vi "Test Refresh Existing Rectangle Settings.vi"(8 "error in (no error)":errorcluster) -> (0 "error out":errorcluster)   [LabVIEW 2019]
uses:
  Setting Database/Setting Database.lvclass
  C:/Program Files (x86)/National Instruments/LabVIEW 2019/vi.lib/JKI/JKI SMO/SMO/SMO.lvclass
  ObjectSettings/ObjectSettings.lvclass/ObjectSettings.ctl
  ObjectSettings/Accessors/Read Enabled.vi
  ObjectSettings/Accessors/Write Enabled.vi
  Rectangle Settings/Rectangle Settings.lvclass
  C:/Users/Albro/Documents/GitHub/AFM-Lithography/lvsrc/Classes/Settings/ObjectSettings/ObjectSettings.lvclass
  <vilib>/addons/_JKI Toolkits/Caraya/classes/Assert/Assert Equal Value_Variant.vi
  <vilib>/addons/_JKI Toolkits/Caraya/classes/Test/Test.lvclass
  <vilib>/addons/_JKI Toolkits/Caraya/classes/Assert/Assert.lvclass
  <vilib>/JKI/JKI SMO/SMO/SMO.lvclass
  <vilib>/LabVIEW Open Source Project/Unicity/RandomStringGenerator/RandomStringGenerator.lvclass
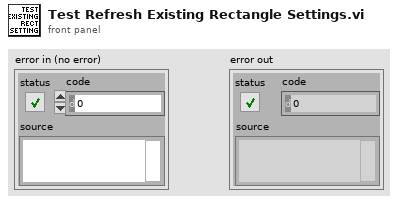
[diagram p1: front panel]
types:
  T1 = typedef "Setting Database.lvclass/PublicEvents--Cluster.ctl" = cluster{"NewActivePath":refnum<user-event>, "PathsUpdated":refnum<user-event>, "RectanglesUpdated":refnum<user-event>, "NewActiveRectangle":refnum<user-event>, "NewActiveFunnel":refnum<user-event>, "FunnelsUpdated":refnum<user-event>, "NewActiveDot":refnum<user-event>, "DotsUpdated":refnum<user-event>}
  T2 = typedef "Setting Database.lvclass/PrivateEvents--Setting Database.Refresh.ctl" = cluster{"Paths":string[], "Rectangles":string[], "Funnels":string[], "Dots":string[]}
  T3 = typedef "Setting Database.lvclass/PublicEvents--Setting Database.NewActiveRectangle.ctl" = refnum<class "Rectangle Settings.lvclass">
  T4 = typedef "Setting Database.lvclass/PublicEvents--Setting Database.RectanglesUpdated.ctl" = refnum<class "Rectangle Settings.lvclass">[]
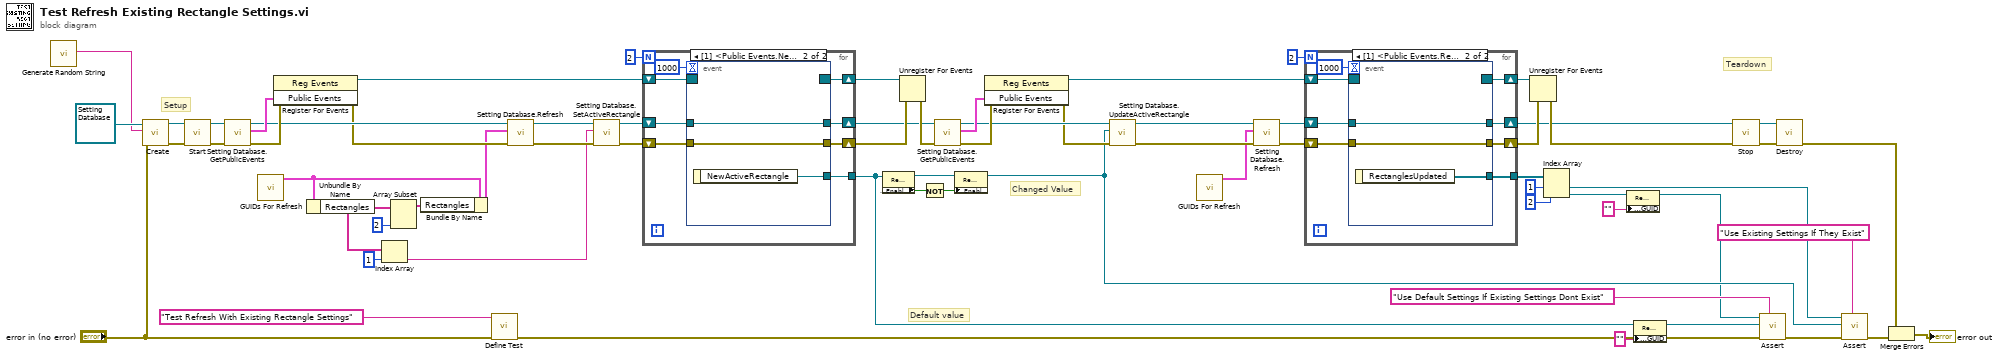
[diagram p0: block diagram]
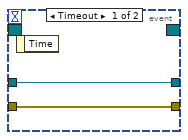
[diagram p2: hidden frame]
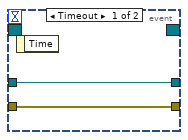
[diagram p3: hidden frame]
diagram:
  # "Changed Value"
  # "Default value"
  # "Teardown"
  # "Setup"
  n1 = call <vilib>:"Generate Random String.vi"() -> ("Random String"=w1:string)  [unwired: 11 in]
  n2 = call <vilib>:"Create.vi"("error in (no error)"="error in (no error)", "Subsystem Name (optional)"=w1, "SMO"=refnum<class "Setting Database.lvclass"> refnum ("Setting Database.lvclass")) -> ("error out"=w66:errorcluster, "SMO out"=w58:refnum<class "Setting Database.lvclass">)  [unwired: 6 in, 1 out]
  n3 = call <vilib>:"Start.vi"("error in (no error)"=w66, "SMO"=w58) -> ("error out"=w65:errorcluster, "SMO out"=w57:refnum<class "Setting Database.lvclass">)  [unwired: 8 in]
  n4 = call "Setting Database.GetPublicEvents.vi"("error in (no error)"=w65, "Setting Database"=w57) -> ("error out"=w63:errorcluster, "Public Events"=w53:T1, "Setting Database out"=w51:refnum<class "Setting Database.lvclass">)  [unwired: 7 in]
  n5 = call "GUIDs For Refresh.vi"() -> ("Initialize"=w13:T2)  [unwired: 11 in]
  n6 = register-events(error in=w63, w53) -> (reference out=w54:refnum<event-registration>, error out=w50:errorcluster)  [unwired: 1 in]
  n7 = Unbundle By Name(w13) -> ("Rectangles"=w11:string[])
  n8 = Index Array(array=w11, index=1) -> (element=w9:string)
  n9 = Array Subset(array=w11, length=2) -> (w14:string[])  [unwired: 1 in]
  n10 = Bundle By Name(cluster=w13, "Rectangles"=w14) -> (w12:T2)
  n11 = call <vilib>:"Define Test.vi"("error in (no error)"="error in (no error)", "Label (VI Title)"="Test Refresh With Existing Rectangle Settings") -> ("error out"=w25:errorcluster)  [unwired: 8 in, 1 out]
  n12 = call "Setting Database.Refresh.vi"("error in (no error)"=w50, "Initialize"=w12, "Setting Database"=w51) -> ("error out"=w21:errorcluster, "Setting Database out"=w24:refnum<class "Setting Database.lvclass">)  [unwired: 7 in]
  n13 = call "Setting Database.SetActiveRectangle.vi"("error in (no error)"=w21, "SetActiveRectangle"=w9, "Setting Database"=w24) -> ("error out"=w22:errorcluster, "Setting Database out"=w23:refnum<class "Setting Database.lvclass">)  [unwired: 7 in]
  n14 = for {
    N: 2 -> [_]
    tunnel: [w68] -> w6
    shift-right: [w74] -> w55
    shift-left: w54 -> [w72]
    shift-right: [w75] -> w45
    shift-left: w22 -> [w70]
    shift-right: [w71] -> w41
    shift-left: w23 -> [w69]
    n15 = event shown="[1] <Public Events.NewActiveRectangle>: User Event" {
      selector: w72 -> [_ _]
      dyn-events: [_ _] -> w74
      timeout: 1000 -> [_ _]
      tunnel: [w77 w80] -> w75
      tunnel: w70 -> [w77 w80]
      tunnel: w69 -> [w76 w79]
      tunnel: [w76 w79] -> w71
      tunnel: [_ w78] -> w68
      event Timeout {
        n16 = event-data() -> ()  [unwired: 1 in, 1 out]
      }
      event User Event {
        n17 = event-data() -> ("NewActiveRectangle"=w78:T3)  [unwired: 1 in]
      }
    }
  }
  n18 = property on="Property Node" class="Rectangle Settings.lvclass"(reference=w6) -> (reference out=w47:T3, "Accessors:Enabled"=w49:bool)  [unwired: 1 in, 1 out]
  n19 = Unregister For Events(event registration refnum=w55, error in=w45) -> (error out=w42:errorcluster)
  n20 = Not(x=w49) -> (.not. x?=w48:bool)
  n21 = call "Setting Database.GetPublicEvents.vi"("error in (no error)"=w42, "Setting Database"=w41) -> ("error out"=w43:errorcluster, "Public Events"=w44:T1, "Setting Database out"=w20:refnum<class "Setting Database.lvclass">)  [unwired: 7 in]
  n22 = property on="Property Node" class="Rectangle Settings.lvclass"(reference=w47, "Accessors:Enabled"=w48) -> (reference out=w16:T3)  [unwired: 1 in, 1 out]
  n23 = register-events(error in=w43, w44) -> (reference out=w38:refnum<event-registration>, error out=w17:errorcluster)  [unwired: 1 in]
  n24 = call "Setting Database.UpdateActiveRectangle.vi"("error in (no error)"=w17, "UpdateActiveRectangle"=w16, "Setting Database"=w20) -> ("error out"=w18:errorcluster, "Setting Database"=w19:refnum<class "Setting Database.lvclass">)  [unwired: 7 in]
  n25 = call "GUIDs For Refresh.vi"() -> ("Initialize"=w8:T2)  [unwired: 11 in]
  n26 = call "Setting Database.Refresh.vi"("error in (no error)"=w18, "Initialize"=w8, "Setting Database"=w19) -> ("error out"=w40:errorcluster, "Setting Database out"=w39:refnum<class "Setting Database.lvclass">)  [unwired: 7 in]
  n27 = for {
    N: 2 -> [_]
    tunnel: [w81] -> w33
    shift-right: [w87] -> w37
    shift-left: w38 -> [w85]
    shift-right: [w88] -> w36
    shift-left: w40 -> [w83]
    shift-right: [w84] -> w34
    shift-left: w39 -> [w82]
    n28 = event shown="[1] <Public Events.RectanglesUpdated>: User Event" {
      selector: w85 -> [_ _]
      dyn-events: [_ _] -> w87
      timeout: 1000 -> [_ _]
      tunnel: [w90 w93] -> w88
      tunnel: w83 -> [w90 w93]
      tunnel: w82 -> [w89 w92]
      tunnel: [w89 w92] -> w84
      tunnel: [_ w91] -> w81
      event Timeout {
        n29 = event-data() -> ()  [unwired: 1 in, 1 out]
      }
      event User Event {
        n30 = event-data() -> ("RectanglesUpdated"=w91:T4)  [unwired: 1 in]
      }
    }
  }
  n31 = Unregister For Events(event registration refnum=w37, error in=w36) -> (error out=w35:errorcluster)
  n32 = Index Array(array=w33, index #1=1 ("index"), index #2=2 ("index")) -> (element #1=w30:refnum<class "Rectangle Settings.lvclass">, element #2=w4:refnum<class "Rectangle Settings.lvclass">)
  n33 = property class="Rectangle Settings.lvclass"(reference=w4, "Accessors:GUID"="" ("GUID")) -> (reference out=w3:refnum<class "Rectangle Settings.lvclass">)  [unwired: 1 in, 1 out]
  n34 = property class="Rectangle Settings.lvclass"(reference=w6, "Accessors:GUID"="" ("GUID")) -> (reference out=w5:T3)  [unwired: 1 in, 1 out]
  n35 = call <vilib>:"Stop.vi"("error in (no error)"=w35, "SMO"=w34) -> ("error out"=w64:errorcluster, "SMO out"=w56:refnum<class "Setting Database.lvclass">)  [unwired: 8 in]
  n36 = call-poly <vilib>:"Assert.vi"("Label"="Use Default Settings If Existing Settings Dont Exist", "error in (no error)"=w25, "Actual"=w5, "Expected"=w3) -> ("error out"=w27:errorcluster)  [unwired: 6 in, 1 out]
  n37 = call <vilib>:"Destroy.vi"("error in (no error)"=w64, "SMO"=w56) -> ("error out"=w62:errorcluster)  [unwired: 9 in]
  n38 = call-poly <vilib>:"Assert.vi"("Label"="Use Existing Settings If They Exist" ("Label (VI Title)"), "error in (no error)"=w27, "Actual"=w16, "Expected"=w30) -> ("error out"=w26:errorcluster)  [unwired: 6 in, 1 out]
  n39 = Merge Errors(w62, w26) -> (→"error out":errorcluster)
